vi "Drive Controller.vi"(8 "error in":errorcluster) -> ()   [LabVIEW 2017]
doc: "This VI executes continuously carrying out the current operation and responding to updates or new operation requests. It will often contain the timing or control code that is difficult to place directly in TeleOp. This VI generally opens all sensors and motors and isolates the rest of the robot code from knowing implementation details of how the operations are carried out."
uses:
  Drive Operations.ctl
  Drive Setpoints.ctl
  <vilib>/Rock Robotics/WPI/SafetyOutput/WPI_SafetyOutputConfigMenu.ctl
  Public/Documents/Cross The Road Electronics/Phoenix-LabVIEW/Motor Controller/Controls/CTRE_Phoenix_MotorControl_ControlMode.ctl
  Public/Documents/Cross The Road Electronics/Phoenix-LabVIEW/Motor Controller/Controls/CTRE_Phoenix_MotorControl_NeutralMode.ctl
  Public/Documents/Cross The Road Electronics/Phoenix-LabVIEW/Motor Controller/Controls/CTRE_Phoenix_MotorControl_FeedbackDevice.ctl
  <vilib>/Rock Robotics/WPI/RobotDrive/WPI_RobotDriveOpen4MotorWithExistingMotors.vi
  <vilib>/Rock Robotics/WPI/RobotDrive/WPI_RobotDriveOpen2MotorWithExistingMotors.vi
  <vilib>/Rock Robotics/WPI/Framework/Completion Status.ctl
panel:
  in  "Interactive Values":T1
  in  "Buttons":cluster{"Execute Cmd":bool, "Abort Cmd":bool}
  out "Command Timing":cluster{"Start Time (ms)":u32, "Iterations":i32}
  out "Status":T3
  out "Setpoints":T4(graph)
  out "Current\nCmd":string
  # "Tip: The graph shows the motor setpoints. It may also be helpful to observe inputs and sensor values.\nYou may also want to display tuning or debugging controls."
  # "Interactive Command: You may fill in the settings for a command\nand schedule it with the Execute button. You can observe and abort\nany command while fine tuning the code for the controller."
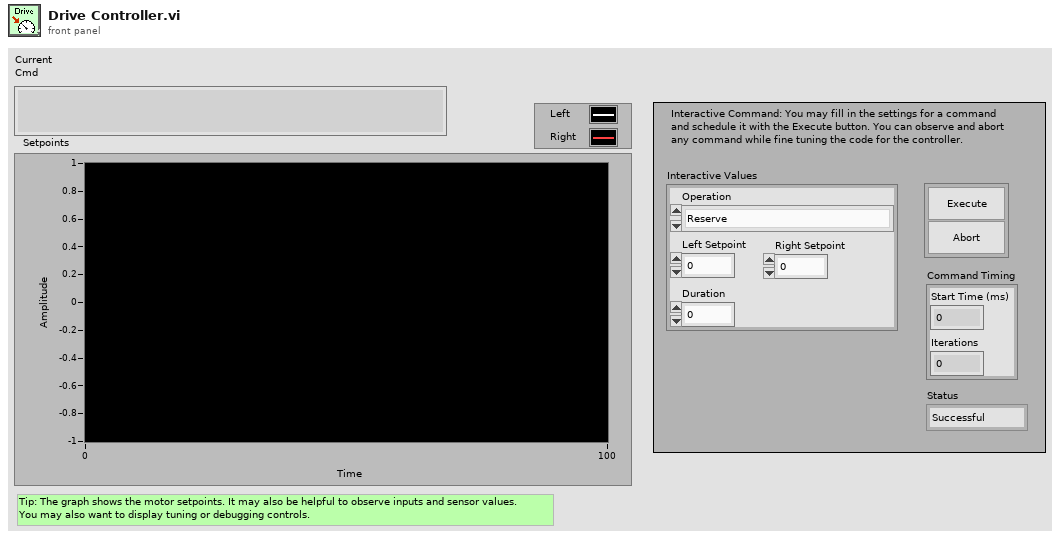
[diagram p1: front panel]
types:
  T1 = typedef "Drive Setpoints.ctl" = cluster{"Operation":T2, "Left Setpoint":dbl, "Right Setpoint":dbl, "Duration":dbl}
  T2 = typedef "Drive Operations.ctl" = enum16{"Reserve", "Read Current", "Immediate", "Drive for Time", "Drive for Distance"}
  T3 = typedef "Completion Status.ctl" = enum16{"Successful", "Aborted", "Incomplete"}
  T4 = cluster{"Left Setpoint":dbl, "Right Setpoint":dbl}
  T5 = typedef "WPI_SafetyOutputConfigMenu.ctl" = enum16{"Enable", "Disable"}
  T6 = typedef "CTRE_Phoenix_MotorControl_NeutralMode.ctl" = enum8{"EEPROMSetting", "Override to Coast", "Override to Brake"}
  T7 = typedef "CTRE_Phoenix_MotorControl_ControlMode.ctl" = u16
  T8 = typedef "CTRE_Phoenix_MotorControl_FeedbackDevice.ctl" = i8
  T9 = typedef "WPI_MotorControlDeviceRef.ctl" = cluster{"DeviceStatus":errorcluster, "Type":T10, "PWM":cluster{"PWM Channel":T11, "DeadBand":T12}, "CAN":cluster{"Device Number":u8, "SetOutput VI Ref":variant, "GetOutput VI Ref":variant, "Enable VI Ref":variant, "Disable VI Ref":variant, "Data":variant}, "Invert":bool, "DIO PWM":cluster{"PWM \"Enable\" Channel":T11, "DIOChannel":T13, "PWM Rate":dbl}}
  T10 = typedef "WPI_MotorControlType.ctl" = enum16{"PWM", "CAN", "DIO PWM"}
  T11 = typedef "FPGA_DIOPWMChannel.ctl" = enum8{"PWM 0", "PWM 1", "PWM 2", "PWM 3", "PWM 4", "PWM 5", "PWM 6", "PWM 7", "PWM 8", "PWM 9", "PWM MXP 0", "PWM MXP 1", "PWM MXP 2", "PWM MXP 3", "PWM MXP 4", "PWM MXP 5", "PWM MXP 6", "PWM MXP 7", "PWM MXP 8", "PWM MXP 9", "Invalid"}
  T12 = typedef "WPI_PWMDeadband.ctl" = cluster{"Name":string, "maxPositivePwm":i32, "minPositivePwm":i32, "centerPwm":i32, "maxNegativePwm":i32, "minNegativePwm":i32, "angularRange":u16}
  T13 = typedef "FPGA_DIOChannel.ctl" = enum8{"DIO 0", "DIO 1", "DIO 2", "DIO 3", "DIO 4", "DIO 5", "DIO 6", "DIO 7", "DIO 8", "DIO 9", "DIO MXP 0", "DIO MXP 1", "DIO MXP 2", "DIO MXP 3", "DIO MXP 4", "DIO MXP 5", "DIO MXP 6", "DIO MXP 7", "DIO MXP 8", "DIO MXP 9", "DIO MXP 10", "DIO MXP 11", "DIO MXP 12", "DIO MXP 13", "DIO MXP 14", "DIO MXP 15", "SPI Port CS1", "SPI Port CS2", "SPI Port CS3", "SPI Port MISO", "SPI Port MOSI", "Invalid"}
  T14 = typedef "WPI_RobotDriveDevRef.ctl" = cluster{"DevStatus":errorcluster, "Motors[]":T9[], "Square Inputs":bool, "Max Output":dbl}
  T15 = typedef "Command Status Info.ctl" = cluster{"Name":string, "Status":T3, "notifier out":T16}
  T16 = typedef "Completion Notifier.ctl" = refnum<notifier>
  T17 = cluster{"SubSystem Data":T1, cluster{"Start Time (ms)":u32, "Iterations":i32}, cluster{"Command Info":T15, "Description":string, "Default Command":T1, "queue out":refnum<queue>, "Subsystem Name":string}}
  T18 = cluster{"SubSystem Data":T1, cluster{"Start Time (ms)":u32, "Iterations":i32}, "Default Command Arguments":cluster{"Command Info":T15, "Description":string, "Default Command":T1, "queue out":refnum<queue>, "Subsystem Name":string}}
  T19 = cluster{"Don't move motors while reserved":dbl, "Don't move motors while reserved":dbl}
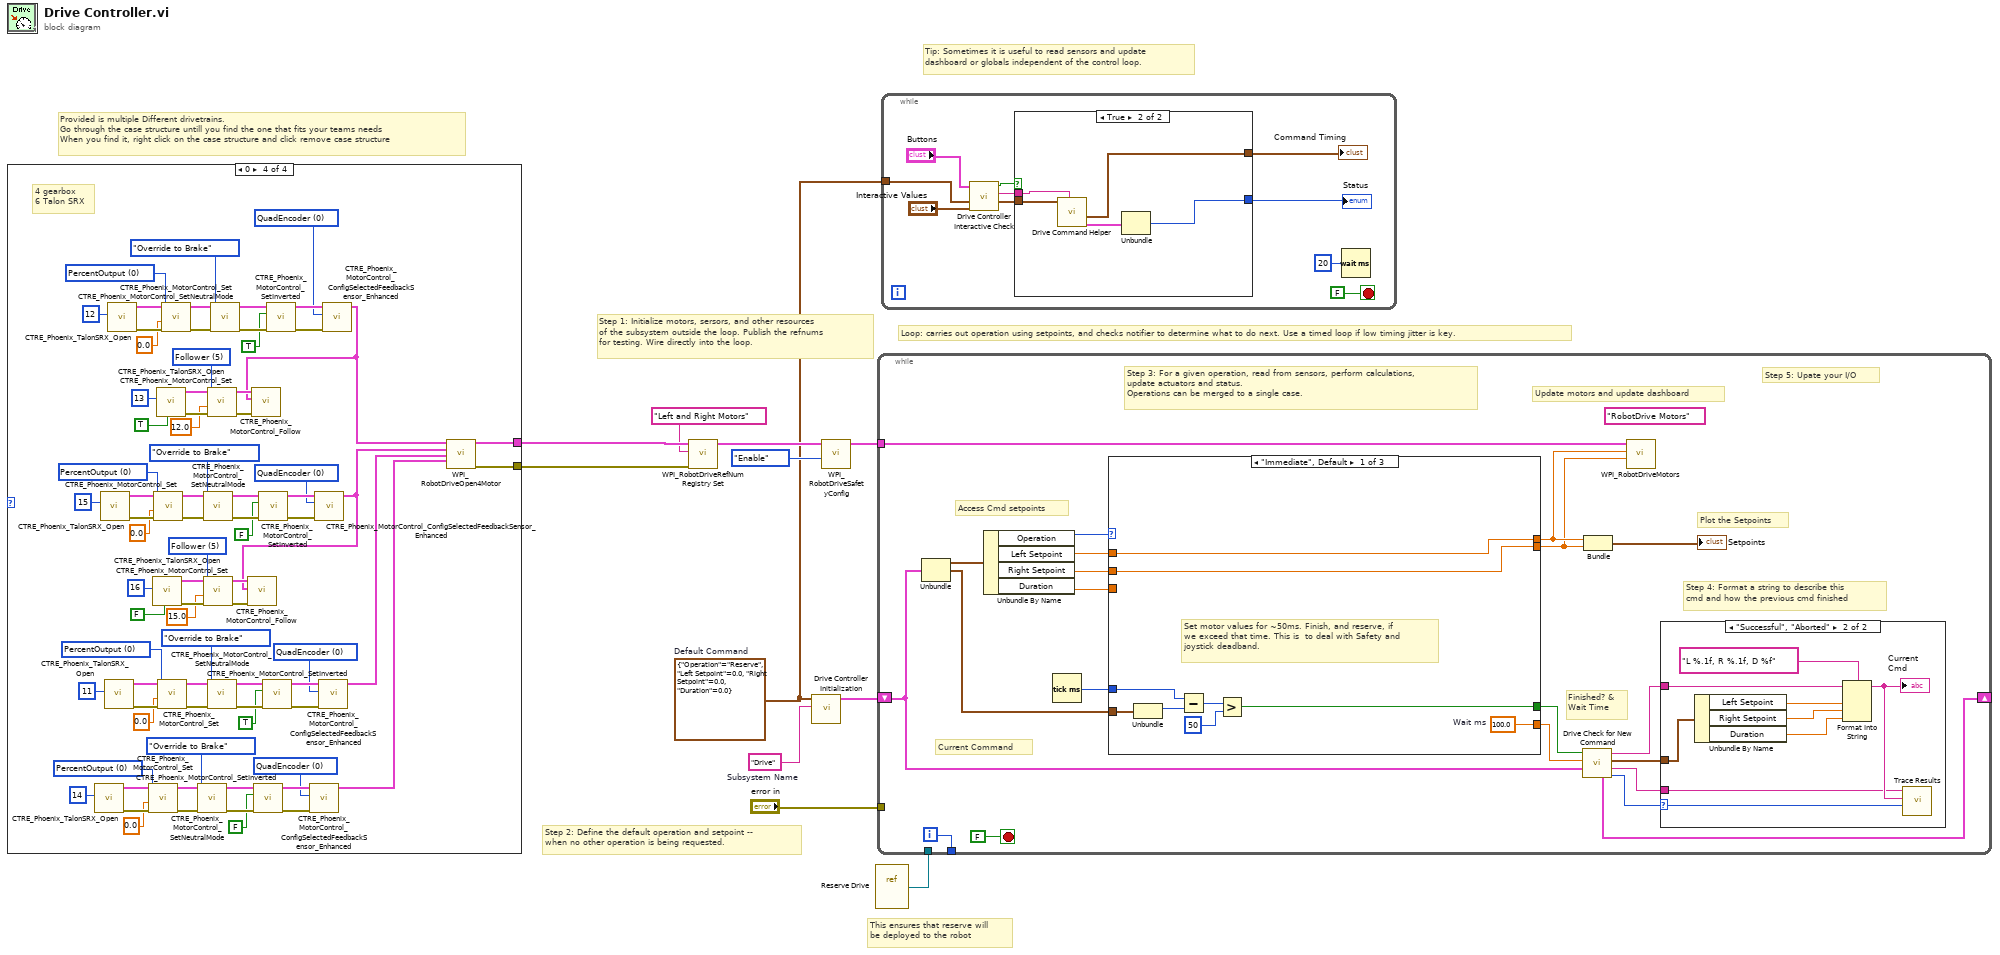
[diagram p0: block diagram]
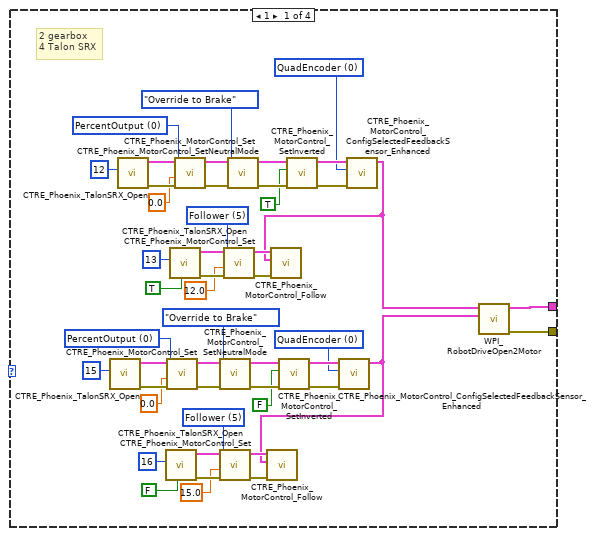
[diagram p2: hidden frame]
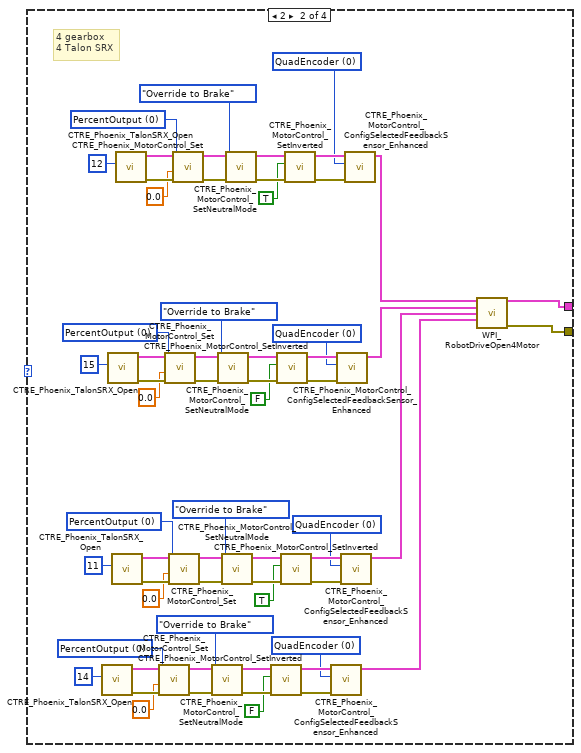
[diagram p3: hidden frame]
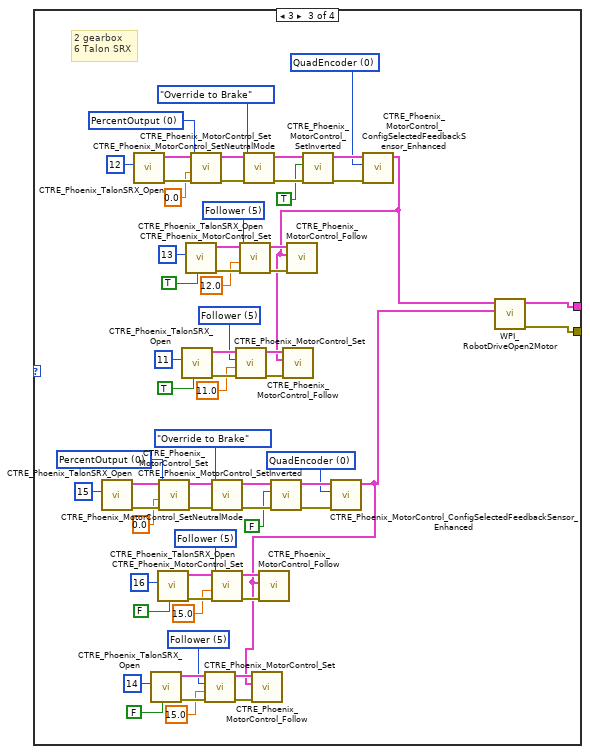
[diagram p4: hidden frame]
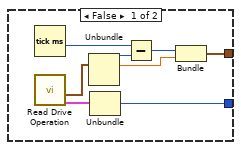
[diagram p5: hidden frame]
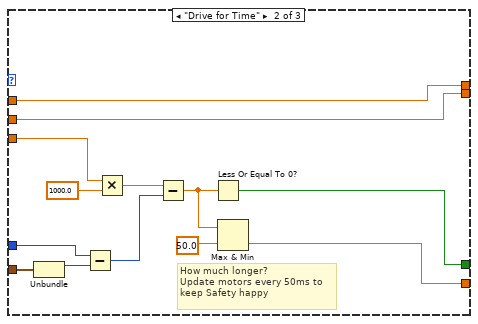
[diagram p7: hidden frame]
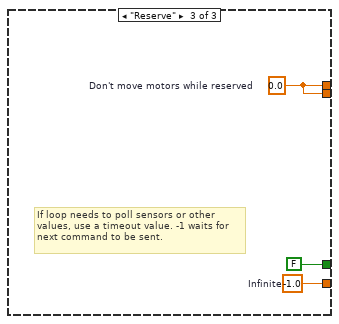
[diagram p8: hidden frame]
diagram:
  w1 = T1 {"Operation"=enum."Reserve", "Left Setpoint"=0.0, "Right Setpoint"=0.0, "Duration"=0.0}  # Default Command
  w11 = "Drive"  # Subsystem Name
  # "Provided is multiple Different drivetrains. \nGo through the case structure untill you find the one that fits your teams needs\nWhen you find it, right click on the case structure and click remove case structure"
  # "This ensures that reserve will\nbe deployed to the robot"
  # "Tip: Sometimes it is useful to read sensors and update\ndashboard or globals independent of the control loop."
  # "Step 2: Define the default operation and setpoint --\nwhen no other operation is being requested."
  # "Step 1: Initialize motors, sersors, and other resources\nof the subsystem outside the loop. Publish the refnums\nfor testing. Wire directly into the loop."
  # "Loop: carries out operation using setpoints, and checks notifier to determine what to do next. Use a timed loop if low timing jitter is key."
  n1 = case shown="0" {
    selector: _ -> [_ _ _ _]
    tunnel: [w15 w61 w141 w263] -> w10
    tunnel: [w14 w60 w140 w262] -> w8
    frame 1 {
      w21 = T7 5 items=["PercentOutput"=0, "Position"=1, "Velocity"=2, "Follower"=5, "MotionProfile"=6, "MotionMagic"=7, "MotionMagicArc"=8, "TimedPercentOutput"=9, "Disabled"=15] ("Control Mode")
      w28 = T7 5 items=["PercentOutput"=0, "Position"=1, "Velocity"=2, "Follower"=5, "MotionProfile"=6, "MotionMagic"=7, "MotionMagicArc"=8, "TimedPercentOutput"=9, "Disabled"=15] ("Control Mode")
      w32 = T8 0 items=["None"=-1, "QuadEncoder"=0, "Analog"=2, "Tachometer"=4, "Pulse Width Encoded Position"=8, "Sensor Sum (S0 + S1)"=9, "Sensor Difference (D0 - D1)"=10, "Remote Source 0"=11, "Remote Source 1"=12, "Software Emulated"=15] ("Feedback Device")
      w43 = T7 0 items=["PercentOutput"=0, "Position"=1, "Velocity"=2, "Follower"=5, "MotionProfile"=6, "MotionMagic"=7, "MotionMagicArc"=8, "TimedPercentOutput"=9, "Disabled"=15] ("Control Mode")
      w46 = T8 0 items=["None"=-1, "QuadEncoder"=0, "Analog"=2, "Tachometer"=4, "Pulse Width Encoded Position"=8, "Sensor Sum (S0 + S1)"=9, "Sensor Difference (D0 - D1)"=10, "Remote Source 0"=11, "Remote Source 1"=12, "Software Emulated"=15] ("Feedback Device")
      w57 = T7 0 items=["PercentOutput"=0, "Position"=1, "Velocity"=2, "Follower"=5, "MotionProfile"=6, "MotionMagic"=7, "MotionMagicArc"=8, "TimedPercentOutput"=9, "Disabled"=15] ("Control Mode")
      # "2 gearbox\n4 Talon SRX"
      n2 = call "CTRE_Phoenix_TalonSRX_Open.vi"("Device Number"=u8 15) -> ("error out"=w45:errorcluster, "CAN Talon SRX Ref"=w44:T9)  [unwired: 9 in]
      n3 = call "CTRE_Phoenix_TalonSRX_Open.vi"("Device Number"=u8 12) -> ("error out"=w59:errorcluster, "CAN Talon SRX Ref"=w58:T9)  [unwired: 9 in]
      n4 = call "CTRE_Phoenix_TalonSRX_Open.vi"("Invert"=FALSE, "Device Number"=u8 16) -> ("error out"=w23:errorcluster, "CAN Talon SRX Ref"=w22:T9)  [unwired: 8 in]
      n5 = call "CTRE_Phoenix_MotorControl_Set.vi"("error in (no error)"=w45, "Output"=0.0, "Control Mode"=w43, "PhoenixMotorControlDevRef"=w44) -> ("error out"=w40:errorcluster, "PhoenixMotorControlDevRef"=w39:T9)  [unwired: 6 in]
      n6 = call "CTRE_Phoenix_TalonSRX_Open.vi"("Invert"=TRUE, "Device Number"=u8 13) -> ("error out"=w30:errorcluster, "CAN Talon SRX Ref"=w29:T9)  [unwired: 8 in]
      n7 = call "CTRE_Phoenix_MotorControl_Set.vi"("error in (no error)"=w59, "Output"=0.0, "Control Mode"=w57, "PhoenixMotorControlDevRef"=w58) -> ("error out"=w54:errorcluster, "PhoenixMotorControlDevRef"=w53:T9)  [unwired: 6 in]
      n8 = call "CTRE_Phoenix_MotorControl_SetNeutralMode.vi"("error in (no error)"=w40, "Motor Control Neutral Mode"=CTRE_Phoenix_MotorControl_NeutralMode."Override to Brake", "PhoenixMotorControlDevRef"=w39) -> ("error out"=w37:errorcluster, "PhoenixMotorControlDevRef"=w36:T9)  [unwired: 7 in]
      n9 = call "CTRE_Phoenix_MotorControl_Set.vi"("error in (no error)"=w23, "Output"=15.0, "Control Mode"=w21, "PhoenixMotorControlDevRef"=w22) -> ("error out"=w19:errorcluster, "PhoenixMotorControlDevRef"=w18:T9)  [unwired: 6 in]
      n10 = call "CTRE_Phoenix_MotorControl_Set.vi"("error in (no error)"=w30, "Output"=12.0, "Control Mode"=w28, "PhoenixMotorControlDevRef"=w29) -> ("error out"=w26:errorcluster, "PhoenixMotorControlDevRef"=w25:T9)  [unwired: 6 in]
      n11 = call "CTRE_Phoenix_MotorControl_SetNeutralMode.vi"("error in (no error)"=w54, "Motor Control Neutral Mode"=CTRE_Phoenix_MotorControl_NeutralMode."Override to Brake", "PhoenixMotorControlDevRef"=w53) -> ("error out"=w51:errorcluster, "PhoenixMotorControlDevRef"=w50:T9)  [unwired: 7 in]
      n12 = call "CTRE_Phoenix_MotorControl_SetInverted.vi"("error in (no error)"=w37, "Invert?"=FALSE, "PhoenixMotorControlDevRef"=w36) -> ("error out"=w34:errorcluster, "PhoenixMotorControlDevRef"=w33:T9)  [unwired: 7 in]
      n13 = call "CTRE_Phoenix_MotorControl_SetInverted.vi"("error in (no error)"=w51, "Invert?"=TRUE, "PhoenixMotorControlDevRef"=w50) -> ("error out"=w48:errorcluster, "PhoenixMotorControlDevRef"=w47:T9)  [unwired: 7 in]
      n14 = call "CTRE_Phoenix_MotorControl_ConfigSelectedFeedbackSensor_Enhanced.vi"("error in (no error)"=w34, "Feedback Device"=w32, "PhoenixMotorControlDevRef"=w33) -> ("PhoenixMotorControlDevRef"=w12:T9)  [unwired: 7 in, 1 out]
      n15 = call "CTRE_Phoenix_MotorControl_Follow.vi"("error in (no error)"=w19, "Master Controller to Follow"=w12, "PhoenixMotorControlDevRef"=w18) -> ()  [unwired: 7 in, 2 out]
      n16 = call "CTRE_Phoenix_MotorControl_ConfigSelectedFeedbackSensor_Enhanced.vi"("error in (no error)"=w48, "Feedback Device"=w46, "PhoenixMotorControlDevRef"=w47) -> ("PhoenixMotorControlDevRef"=w13:T9)  [unwired: 7 in, 1 out]
      n17 = call "CTRE_Phoenix_MotorControl_Follow.vi"("error in (no error)"=w26, "Master Controller to Follow"=w13, "PhoenixMotorControlDevRef"=w25) -> ()  [unwired: 7 in, 2 out]
      n18 = call-poly <vilib>:"WPI_RobotDriveOpen2Motor.vi"("Right Motor Dev Ref"=w12, "Left Motor Dev Ref"=w13) -> ("error out"=w14:errorcluster, "RobotDriveDevRef"=w15:T14)  [unwired: 8 in]
    }
    frame 2 {
      w66 = T8 0 items=["None"=-1, "QuadEncoder"=0, "Analog"=2, "Tachometer"=4, "Pulse Width Encoded Position"=8, "Sensor Sum (S0 + S1)"=9, "Sensor Difference (D0 - D1)"=10, "Remote Source 0"=11, "Remote Source 1"=12, "Software Emulated"=15] ("Feedback Device")
      w77 = T7 0 items=["PercentOutput"=0, "Position"=1, "Velocity"=2, "Follower"=5, "MotionProfile"=6, "MotionMagic"=7, "MotionMagicArc"=8, "TimedPercentOutput"=9, "Disabled"=15] ("Control Mode")
      w80 = T8 0 items=["None"=-1, "QuadEncoder"=0, "Analog"=2, "Tachometer"=4, "Pulse Width Encoded Position"=8, "Sensor Sum (S0 + S1)"=9, "Sensor Difference (D0 - D1)"=10, "Remote Source 0"=11, "Remote Source 1"=12, "Software Emulated"=15] ("Feedback Device")
      w91 = T7 0 items=["PercentOutput"=0, "Position"=1, "Velocity"=2, "Follower"=5, "MotionProfile"=6, "MotionMagic"=7, "MotionMagicArc"=8, "TimedPercentOutput"=9, "Disabled"=15] ("Control Mode")
      w94 = T8 0 items=["None"=-1, "QuadEncoder"=0, "Analog"=2, "Tachometer"=4, "Pulse Width Encoded Position"=8, "Sensor Sum (S0 + S1)"=9, "Sensor Difference (D0 - D1)"=10, "Remote Source 0"=11, "Remote Source 1"=12, "Software Emulated"=15] ("Feedback Device")
      w105 = T7 0 items=["PercentOutput"=0, "Position"=1, "Velocity"=2, "Follower"=5, "MotionProfile"=6, "MotionMagic"=7, "MotionMagicArc"=8, "TimedPercentOutput"=9, "Disabled"=15] ("Control Mode")
      w108 = T8 0 items=["None"=-1, "QuadEncoder"=0, "Analog"=2, "Tachometer"=4, "Pulse Width Encoded Position"=8, "Sensor Sum (S0 + S1)"=9, "Sensor Difference (D0 - D1)"=10, "Remote Source 0"=11, "Remote Source 1"=12, "Software Emulated"=15] ("Feedback Device")
      w119 = T7 0 items=["PercentOutput"=0, "Position"=1, "Velocity"=2, "Follower"=5, "MotionProfile"=6, "MotionMagic"=7, "MotionMagicArc"=8, "TimedPercentOutput"=9, "Disabled"=15] ("Control Mode")
      # "4 gearbox\n4 Talon SRX"
      n19 = call "CTRE_Phoenix_TalonSRX_Open.vi"("Device Number"=u8 14) -> ("error out"=w79:errorcluster, "CAN Talon SRX Ref"=w78:T9)  [unwired: 9 in]
      n20 = call "CTRE_Phoenix_TalonSRX_Open.vi"("Device Number"=u8 15) -> ("error out"=w107:errorcluster, "CAN Talon SRX Ref"=w106:T9)  [unwired: 9 in]
      n21 = call "CTRE_Phoenix_TalonSRX_Open.vi"("Device Number"=u8 11) -> ("error out"=w93:errorcluster, "CAN Talon SRX Ref"=w92:T9)  [unwired: 9 in]
      n22 = call "CTRE_Phoenix_TalonSRX_Open.vi"("Device Number"=u8 12) -> ("error out"=w121:errorcluster, "CAN Talon SRX Ref"=w120:T9)  [unwired: 9 in]
      n23 = call "CTRE_Phoenix_MotorControl_Set.vi"("error in (no error)"=w79, "Output"=0.0, "Control Mode"=w77, "PhoenixMotorControlDevRef"=w78) -> ("error out"=w74:errorcluster, "PhoenixMotorControlDevRef"=w73:T9)  [unwired: 6 in]
      n24 = call "CTRE_Phoenix_MotorControl_Set.vi"("error in (no error)"=w107, "Output"=0.0, "Control Mode"=w105, "PhoenixMotorControlDevRef"=w106) -> ("error out"=w102:errorcluster, "PhoenixMotorControlDevRef"=w101:T9)  [unwired: 6 in]
      n25 = call "CTRE_Phoenix_MotorControl_Set.vi"("error in (no error)"=w93, "Output"=0.0, "Control Mode"=w91, "PhoenixMotorControlDevRef"=w92) -> ("error out"=w88:errorcluster, "PhoenixMotorControlDevRef"=w87:T9)  [unwired: 6 in]
      n26 = call "CTRE_Phoenix_MotorControl_Set.vi"("error in (no error)"=w121, "Output"=0.0, "Control Mode"=w119, "PhoenixMotorControlDevRef"=w120) -> ("error out"=w116:errorcluster, "PhoenixMotorControlDevRef"=w115:T9)  [unwired: 6 in]
      n27 = call "CTRE_Phoenix_MotorControl_SetNeutralMode.vi"("error in (no error)"=w74, "Motor Control Neutral Mode"=CTRE_Phoenix_MotorControl_NeutralMode."Override to Brake", "PhoenixMotorControlDevRef"=w73) -> ("error out"=w71:errorcluster, "PhoenixMotorControlDevRef"=w70:T9)  [unwired: 7 in]
      n28 = call "CTRE_Phoenix_MotorControl_SetNeutralMode.vi"("error in (no error)"=w102, "Motor Control Neutral Mode"=CTRE_Phoenix_MotorControl_NeutralMode."Override to Brake", "PhoenixMotorControlDevRef"=w101) -> ("error out"=w99:errorcluster, "PhoenixMotorControlDevRef"=w98:T9)  [unwired: 7 in]
      n29 = call "CTRE_Phoenix_MotorControl_SetNeutralMode.vi"("error in (no error)"=w88, "Motor Control Neutral Mode"=CTRE_Phoenix_MotorControl_NeutralMode."Override to Brake", "PhoenixMotorControlDevRef"=w87) -> ("error out"=w85:errorcluster, "PhoenixMotorControlDevRef"=w84:T9)  [unwired: 7 in]
      n30 = call "CTRE_Phoenix_MotorControl_SetNeutralMode.vi"("error in (no error)"=w116, "Motor Control Neutral Mode"=CTRE_Phoenix_MotorControl_NeutralMode."Override to Brake", "PhoenixMotorControlDevRef"=w115) -> ("error out"=w113:errorcluster, "PhoenixMotorControlDevRef"=w112:T9)  [unwired: 7 in]
      n31 = call "CTRE_Phoenix_MotorControl_SetInverted.vi"("error in (no error)"=w71, "Invert?"=FALSE, "PhoenixMotorControlDevRef"=w70) -> ("error out"=w68:errorcluster, "PhoenixMotorControlDevRef"=w67:T9)  [unwired: 7 in]
      n32 = call "CTRE_Phoenix_MotorControl_SetInverted.vi"("error in (no error)"=w99, "Invert?"=FALSE, "PhoenixMotorControlDevRef"=w98) -> ("error out"=w96:errorcluster, "PhoenixMotorControlDevRef"=w95:T9)  [unwired: 7 in]
      n33 = call "CTRE_Phoenix_MotorControl_SetInverted.vi"("error in (no error)"=w85, "Invert?"=TRUE, "PhoenixMotorControlDevRef"=w84) -> ("error out"=w82:errorcluster, "PhoenixMotorControlDevRef"=w81:T9)  [unwired: 7 in]
      n34 = call "CTRE_Phoenix_MotorControl_SetInverted.vi"("error in (no error)"=w113, "Invert?"=TRUE, "PhoenixMotorControlDevRef"=w112) -> ("error out"=w110:errorcluster, "PhoenixMotorControlDevRef"=w109:T9)  [unwired: 7 in]
      n35 = call "CTRE_Phoenix_MotorControl_ConfigSelectedFeedbackSensor_Enhanced.vi"("error in (no error)"=w68, "Feedback Device"=w66, "PhoenixMotorControlDevRef"=w67) -> ("PhoenixMotorControlDevRef"=w62:T9)  [unwired: 7 in, 1 out]
      n36 = call "CTRE_Phoenix_MotorControl_ConfigSelectedFeedbackSensor_Enhanced.vi"("error in (no error)"=w96, "Feedback Device"=w94, "PhoenixMotorControlDevRef"=w95) -> ("PhoenixMotorControlDevRef"=w64:T9)  [unwired: 7 in, 1 out]
      n37 = call "CTRE_Phoenix_MotorControl_ConfigSelectedFeedbackSensor_Enhanced.vi"("error in (no error)"=w82, "Feedback Device"=w80, "PhoenixMotorControlDevRef"=w81) -> ("PhoenixMotorControlDevRef"=w63:T9)  [unwired: 7 in, 1 out]
      n38 = call "CTRE_Phoenix_MotorControl_ConfigSelectedFeedbackSensor_Enhanced.vi"("error in (no error)"=w110, "Feedback Device"=w108, "PhoenixMotorControlDevRef"=w109) -> ("PhoenixMotorControlDevRef"=w65:T9)  [unwired: 7 in, 1 out]
      n39 = call-poly <vilib>:"WPI_RobotDriveOpen4Motor.vi"("Rear Left Motor Dev Ref"=w65, "Rear Right Motor Dev Ref"=w64, "Front Left Motor Dev Ref"=w63, "Front Right Motor Dev Ref"=w62) -> ("RobotDriveDevRef"=w61:T14, "error out"=w60:errorcluster)  [unwired: 10 in]
    }
    frame 3 {
      w124 = T7 5 items=["PercentOutput"=0, "Position"=1, "Velocity"=2, "Follower"=5, "MotionProfile"=6, "MotionMagic"=7, "MotionMagicArc"=8, "TimedPercentOutput"=9, "Disabled"=15] ("Control Mode")
      w125 = T7 5 items=["PercentOutput"=0, "Position"=1, "Velocity"=2, "Follower"=5, "MotionProfile"=6, "MotionMagic"=7, "MotionMagicArc"=8, "TimedPercentOutput"=9, "Disabled"=15] ("Control Mode")
      w147 = T7 5 items=["PercentOutput"=0, "Position"=1, "Velocity"=2, "Follower"=5, "MotionProfile"=6, "MotionMagic"=7, "MotionMagicArc"=8, "TimedPercentOutput"=9, "Disabled"=15] ("Control Mode")
      w154 = T7 5 items=["PercentOutput"=0, "Position"=1, "Velocity"=2, "Follower"=5, "MotionProfile"=6, "MotionMagic"=7, "MotionMagicArc"=8, "TimedPercentOutput"=9, "Disabled"=15] ("Control Mode")
      w158 = T8 0 items=["None"=-1, "QuadEncoder"=0, "Analog"=2, "Tachometer"=4, "Pulse Width Encoded Position"=8, "Sensor Sum (S0 + S1)"=9, "Sensor Difference (D0 - D1)"=10, "Remote Source 0"=11, "Remote Source 1"=12, "Software Emulated"=15] ("Feedback Device")
      w169 = T7 0 items=["PercentOutput"=0, "Position"=1, "Velocity"=2, "Follower"=5, "MotionProfile"=6, "MotionMagic"=7, "MotionMagicArc"=8, "TimedPercentOutput"=9, "Disabled"=15] ("Control Mode")
      w172 = T8 0 items=["None"=-1, "QuadEncoder"=0, "Analog"=2, "Tachometer"=4, "Pulse Width Encoded Position"=8, "Sensor Sum (S0 + S1)"=9, "Sensor Difference (D0 - D1)"=10, "Remote Source 0"=11, "Remote Source 1"=12, "Software Emulated"=15] ("Feedback Device")
      w183 = T7 0 items=["PercentOutput"=0, "Position"=1, "Velocity"=2, "Follower"=5, "MotionProfile"=6, "MotionMagic"=7, "MotionMagicArc"=8, "TimedPercentOutput"=9, "Disabled"=15] ("Control Mode")
      # "2 gearbox\n6 Talon SRX"
      n40 = call "CTRE_Phoenix_TalonSRX_Open.vi"("Device Number"=u8 15) -> ("error out"=w171:errorcluster, "CAN Talon SRX Ref"=w170:T9)  [unwired: 9 in]
      n41 = call "CTRE_Phoenix_TalonSRX_Open.vi"("Device Number"=u8 12) -> ("error out"=w185:errorcluster, "CAN Talon SRX Ref"=w184:T9)  [unwired: 9 in]
      n42 = call "CTRE_Phoenix_TalonSRX_Open.vi"("Invert"=FALSE, "Device Number"=u8 14) -> ("error out"=w138:errorcluster, "CAN Talon SRX Ref"=w137:T9)  [unwired: 8 in]
      n43 = call "CTRE_Phoenix_TalonSRX_Open.vi"("Invert"=FALSE, "Device Number"=u8 16) -> ("error out"=w149:errorcluster, "CAN Talon SRX Ref"=w148:T9)  [unwired: 8 in]
      n44 = call "CTRE_Phoenix_MotorControl_Set.vi"("error in (no error)"=w171, "Output"=0.0, "Control Mode"=w169, "PhoenixMotorControlDevRef"=w170) -> ("error out"=w166:errorcluster, "PhoenixMotorControlDevRef"=w165:T9)  [unwired: 6 in]
      n45 = call "CTRE_Phoenix_TalonSRX_Open.vi"("Invert"=TRUE, "Device Number"=u8 11) -> ("error out"=w131:errorcluster, "CAN Talon SRX Ref"=w130:T9)  [unwired: 8 in]
      n46 = call "CTRE_Phoenix_TalonSRX_Open.vi"("Invert"=TRUE, "Device Number"=u8 13) -> ("error out"=w156:errorcluster, "CAN Talon SRX Ref"=w155:T9)  [unwired: 8 in]
      n47 = call "CTRE_Phoenix_MotorControl_Set.vi"("error in (no error)"=w185, "Output"=0.0, "Control Mode"=w183, "PhoenixMotorControlDevRef"=w184) -> ("error out"=w180:errorcluster, "PhoenixMotorControlDevRef"=w179:T9)  [unwired: 6 in]
      n48 = call "CTRE_Phoenix_MotorControl_Set.vi"("error in (no error)"=w138, "Output"=15.0, "Control Mode"=w125, "PhoenixMotorControlDevRef"=w137) -> ("error out"=w135:errorcluster, "PhoenixMotorControlDevRef"=w134:T9)  [unwired: 6 in]
      n49 = call "CTRE_Phoenix_MotorControl_SetNeutralMode.vi"("error in (no error)"=w166, "Motor Control Neutral Mode"=CTRE_Phoenix_MotorControl_NeutralMode."Override to Brake", "PhoenixMotorControlDevRef"=w165) -> ("error out"=w163:errorcluster, "PhoenixMotorControlDevRef"=w162:T9)  [unwired: 7 in]
      n50 = call "CTRE_Phoenix_MotorControl_Set.vi"("error in (no error)"=w149, "Output"=15.0, "Control Mode"=w147, "PhoenixMotorControlDevRef"=w148) -> ("error out"=w145:errorcluster, "PhoenixMotorControlDevRef"=w144:T9)  [unwired: 6 in]
      n51 = call "CTRE_Phoenix_MotorControl_Set.vi"("error in (no error)"=w131, "Output"=11.0, "Control Mode"=w124, "PhoenixMotorControlDevRef"=w130) -> ("error out"=w128:errorcluster, "PhoenixMotorControlDevRef"=w127:T9)  [unwired: 6 in]
      n52 = call "CTRE_Phoenix_MotorControl_Set.vi"("error in (no error)"=w156, "Output"=12.0, "Control Mode"=w154, "PhoenixMotorControlDevRef"=w155) -> ("error out"=w152:errorcluster, "PhoenixMotorControlDevRef"=w151:T9)  [unwired: 6 in]
      n53 = call "CTRE_Phoenix_MotorControl_SetNeutralMode.vi"("error in (no error)"=w180, "Motor Control Neutral Mode"=CTRE_Phoenix_MotorControl_NeutralMode."Override to Brake", "PhoenixMotorControlDevRef"=w179) -> ("error out"=w177:errorcluster, "PhoenixMotorControlDevRef"=w176:T9)  [unwired: 7 in]
      n54 = call "CTRE_Phoenix_MotorControl_SetInverted.vi"("error in (no error)"=w163, "Invert?"=FALSE, "PhoenixMotorControlDevRef"=w162) -> ("error out"=w160:errorcluster, "PhoenixMotorControlDevRef"=w159:T9)  [unwired: 7 in]
      n55 = call "CTRE_Phoenix_MotorControl_SetInverted.vi"("error in (no error)"=w177, "Invert?"=TRUE, "PhoenixMotorControlDevRef"=w176) -> ("error out"=w174:errorcluster, "PhoenixMotorControlDevRef"=w173:T9)  [unwired: 7 in]
      n56 = call "CTRE_Phoenix_MotorControl_ConfigSelectedFeedbackSensor_Enhanced.vi"("error in (no error)"=w160, "Feedback Device"=w158, "PhoenixMotorControlDevRef"=w159) -> ("PhoenixMotorControlDevRef"=w122:T9)  [unwired: 7 in, 1 out]
      n57 = call "CTRE_Phoenix_MotorControl_Follow.vi"("error in (no error)"=w135, "Master Controller to Follow"=w122, "PhoenixMotorControlDevRef"=w134) -> ()  [unwired: 7 in, 2 out]
      n58 = call "CTRE_Phoenix_MotorControl_Follow.vi"("error in (no error)"=w145, "Master Controller to Follow"=w122, "PhoenixMotorControlDevRef"=w144) -> ()  [unwired: 7 in, 2 out]
      n59 = call "CTRE_Phoenix_MotorControl_ConfigSelectedFeedbackSensor_Enhanced.vi"("error in (no error)"=w174, "Feedback Device"=w172, "PhoenixMotorControlDevRef"=w173) -> ("PhoenixMotorControlDevRef"=w123:T9)  [unwired: 7 in, 1 out]
      n60 = call "CTRE_Phoenix_MotorControl_Follow.vi"("error in (no error)"=w128, "Master Controller to Follow"=w123, "PhoenixMotorControlDevRef"=w127) -> ()  [unwired: 7 in, 2 out]
      n61 = call "CTRE_Phoenix_MotorControl_Follow.vi"("error in (no error)"=w152, "Master Controller to Follow"=w123, "PhoenixMotorControlDevRef"=w151) -> ()  [unwired: 7 in, 2 out]
      n62 = call-poly <vilib>:"WPI_RobotDriveOpen2Motor.vi"("Right Motor Dev Ref"=w122, "Left Motor Dev Ref"=w123) -> ("error out"=w140:errorcluster, "RobotDriveDevRef"=w141:T14)  [unwired: 8 in]
    }
    frame 0 {
      w195 = T7 5 items=["PercentOutput"=0, "Position"=1, "Velocity"=2, "Follower"=5, "MotionProfile"=6, "MotionMagic"=7, "MotionMagicArc"=8, "TimedPercentOutput"=9, "Disabled"=15] ("Control Mode")
      w202 = T7 5 items=["PercentOutput"=0, "Position"=1, "Velocity"=2, "Follower"=5, "MotionProfile"=6, "MotionMagic"=7, "MotionMagicArc"=8, "TimedPercentOutput"=9, "Disabled"=15] ("Control Mode")
      w206 = T8 0 items=["None"=-1, "QuadEncoder"=0, "Analog"=2, "Tachometer"=4, "Pulse Width Encoded Position"=8, "Sensor Sum (S0 + S1)"=9, "Sensor Difference (D0 - D1)"=10, "Remote Source 0"=11, "Remote Source 1"=12, "Software Emulated"=15] ("Feedback Device")
      w217 = T7 0 items=["PercentOutput"=0, "Position"=1, "Velocity"=2, "Follower"=5, "MotionProfile"=6, "MotionMagic"=7, "MotionMagicArc"=8, "TimedPercentOutput"=9, "Disabled"=15] ("Control Mode")
      w220 = T8 0 items=["None"=-1, "QuadEncoder"=0, "Analog"=2, "Tachometer"=4, "Pulse Width Encoded Position"=8, "Sensor Sum (S0 + S1)"=9, "Sensor Difference (D0 - D1)"=10, "Remote Source 0"=11, "Remote Source 1"=12, "Software Emulated"=15] ("Feedback Device")
      w231 = T7 0 items=["PercentOutput"=0, "Position"=1, "Velocity"=2, "Follower"=5, "MotionProfile"=6, "MotionMagic"=7, "MotionMagicArc"=8, "TimedPercentOutput"=9, "Disabled"=15] ("Control Mode")
      w234 = T8 0 items=["None"=-1, "QuadEncoder"=0, "Analog"=2, "Tachometer"=4, "Pulse Width Encoded Position"=8, "Sensor Sum (S0 + S1)"=9, "Sensor Difference (D0 - D1)"=10, "Remote Source 0"=11, "Remote Source 1"=12, "Software Emulated"=15] ("Feedback Device")
      w245 = T7 0 items=["PercentOutput"=0, "Position"=1, "Velocity"=2, "Follower"=5, "MotionProfile"=6, "MotionMagic"=7, "MotionMagicArc"=8, "TimedPercentOutput"=9, "Disabled"=15] ("Control Mode")
      w248 = T8 0 items=["None"=-1, "QuadEncoder"=0, "Analog"=2, "Tachometer"=4, "Pulse Width Encoded Position"=8, "Sensor Sum (S0 + S1)"=9, "Sensor Difference (D0 - D1)"=10, "Remote Source 0"=11, "Remote Source 1"=12, "Software Emulated"=15] ("Feedback Device")
      w259 = T7 0 items=["PercentOutput"=0, "Position"=1, "Velocity"=2, "Follower"=5, "MotionProfile"=6, "MotionMagic"=7, "MotionMagicArc"=8, "TimedPercentOutput"=9, "Disabled"=15] ("Control Mode")
      # "4 gearbox\n6 Talon SRX"
      n63 = call "CTRE_Phoenix_TalonSRX_Open.vi"("Device Number"=u8 14) -> ("error out"=w219:errorcluster, "CAN Talon SRX Ref"=w218:T9)  [unwired: 9 in]
      n64 = call "CTRE_Phoenix_TalonSRX_Open.vi"("Device Number"=u8 15) -> ("error out"=w247:errorcluster, "CAN Talon SRX Ref"=w246:T9)  [unwired: 9 in]
      n65 = call "CTRE_Phoenix_TalonSRX_Open.vi"("Device Number"=u8 11) -> ("error out"=w233:errorcluster, "CAN Talon SRX Ref"=w232:T9)  [unwired: 9 in]
      n66 = call "CTRE_Phoenix_TalonSRX_Open.vi"("Device Number"=u8 12) -> ("error out"=w261:errorcluster, "CAN Talon SRX Ref"=w260:T9)  [unwired: 9 in]
      n67 = call "CTRE_Phoenix_MotorControl_Set.vi"("error in (no error)"=w219, "Output"=0.0, "Control Mode"=w217, "PhoenixMotorControlDevRef"=w218) -> ("error out"=w214:errorcluster, "PhoenixMotorControlDevRef"=w213:T9)  [unwired: 6 in]
      n68 = call "CTRE_Phoenix_TalonSRX_Open.vi"("Invert"=FALSE, "Device Number"=u8 16) -> ("error out"=w197:errorcluster, "CAN Talon SRX Ref"=w196:T9)  [unwired: 8 in]
      n69 = call "CTRE_Phoenix_MotorControl_Set.vi"("error in (no error)"=w247, "Output"=0.0, "Control Mode"=w245, "PhoenixMotorControlDevRef"=w246) -> ("error out"=w242:errorcluster, "PhoenixMotorControlDevRef"=w241:T9)  [unwired: 6 in]
      n70 = call "CTRE_Phoenix_TalonSRX_Open.vi"("Invert"=TRUE, "Device Number"=u8 13) -> ("error out"=w204:errorcluster, "CAN Talon SRX Ref"=w203:T9)  [unwired: 8 in]
      n71 = call "CTRE_Phoenix_MotorControl_Set.vi"("error in (no error)"=w233, "Output"=0.0, "Control Mode"=w231, "PhoenixMotorControlDevRef"=w232) -> ("error out"=w228:errorcluster, "PhoenixMotorControlDevRef"=w227:T9)  [unwired: 6 in]
      n72 = call "CTRE_Phoenix_MotorControl_Set.vi"("error in (no error)"=w261, "Output"=0.0, "Control Mode"=w259, "PhoenixMotorControlDevRef"=w260) -> ("error out"=w256:errorcluster, "PhoenixMotorControlDevRef"=w255:T9)  [unwired: 6 in]
      n73 = call "CTRE_Phoenix_MotorControl_SetNeutralMode.vi"("error in (no error)"=w214, "Motor Control Neutral Mode"=CTRE_Phoenix_MotorControl_NeutralMode."Override to Brake", "PhoenixMotorControlDevRef"=w213) -> ("error out"=w211:errorcluster, "PhoenixMotorControlDevRef"=w210:T9)  [unwired: 7 in]
      n74 = call "CTRE_Phoenix_MotorControl_SetNeutralMode.vi"("error in (no error)"=w242, "Motor Control Neutral Mode"=CTRE_Phoenix_MotorControl_NeutralMode."Override to Brake", "PhoenixMotorControlDevRef"=w241) -> ("error out"=w239:errorcluster, "PhoenixMotorControlDevRef"=w238:T9)  [unwired: 7 in]
      n75 = call "CTRE_Phoenix_MotorControl_Set.vi"("error in (no error)"=w197, "Output"=15.0, "Control Mode"=w195, "PhoenixMotorControlDevRef"=w196) -> ("error out"=w193:errorcluster, "PhoenixMotorControlDevRef"=w192:T9)  [unwired: 6 in]
      n76 = call "CTRE_Phoenix_MotorControl_Set.vi"("error in (no error)"=w204, "Output"=12.0, "Control Mode"=w202, "PhoenixMotorControlDevRef"=w203) -> ("error out"=w200:errorcluster, "PhoenixMotorControlDevRef"=w199:T9)  [unwired: 6 in]
      n77 = call "CTRE_Phoenix_MotorControl_SetNeutralMode.vi"("error in (no error)"=w228, "Motor Control Neutral Mode"=CTRE_Phoenix_MotorControl_NeutralMode."Override to Brake", "PhoenixMotorControlDevRef"=w227) -> ("error out"=w225:errorcluster, "PhoenixMotorControlDevRef"=w224:T9)  [unwired: 7 in]
      n78 = call "CTRE_Phoenix_MotorControl_SetNeutralMode.vi"("error in (no error)"=w256, "Motor Control Neutral Mode"=CTRE_Phoenix_MotorControl_NeutralMode."Override to Brake", "PhoenixMotorControlDevRef"=w255) -> ("error out"=w253:errorcluster, "PhoenixMotorControlDevRef"=w252:T9)  [unwired: 7 in]
      n79 = call "CTRE_Phoenix_MotorControl_SetInverted.vi"("error in (no error)"=w211, "Invert?"=FALSE, "PhoenixMotorControlDevRef"=w210) -> ("error out"=w208:errorcluster, "PhoenixMotorControlDevRef"=w207:T9)  [unwired: 7 in]
      n80 = call "CTRE_Phoenix_MotorControl_SetInverted.vi"("error in (no error)"=w239, "Invert?"=FALSE, "PhoenixMotorControlDevRef"=w238) -> ("error out"=w236:errorcluster, "PhoenixMotorControlDevRef"=w235:T9)  [unwired: 7 in]
      n81 = call "CTRE_Phoenix_MotorControl_SetInverted.vi"("error in (no error)"=w225, "Invert?"=TRUE, "PhoenixMotorControlDevRef"=w224) -> ("error out"=w222:errorcluster, "PhoenixMotorControlDevRef"=w221:T9)  [unwired: 7 in]
      n82 = call "CTRE_Phoenix_MotorControl_SetInverted.vi"("error in (no error)"=w253, "Invert?"=TRUE, "PhoenixMotorControlDevRef"=w252) -> ("error out"=w250:errorcluster, "PhoenixMotorControlDevRef"=w249:T9)  [unwired: 7 in]
      n83 = call "CTRE_Phoenix_MotorControl_ConfigSelectedFeedbackSensor_Enhanced.vi"("error in (no error)"=w208, "Feedback Device"=w206, "PhoenixMotorControlDevRef"=w207) -> ("PhoenixMotorControlDevRef"=w186:T9)  [unwired: 7 in, 1 out]
      n84 = call "CTRE_Phoenix_MotorControl_ConfigSelectedFeedbackSensor_Enhanced.vi"("error in (no error)"=w236, "Feedback Device"=w234, "PhoenixMotorControlDevRef"=w235) -> ("PhoenixMotorControlDevRef"=w188:T9)  [unwired: 7 in, 1 out]
      n85 = call "CTRE_Phoenix_MotorControl_Follow.vi"("error in (no error)"=w193, "Master Controller to Follow"=w188, "PhoenixMotorControlDevRef"=w192) -> ()  [unwired: 7 in, 2 out]
      n86 = call "CTRE_Phoenix_MotorControl_ConfigSelectedFeedbackSensor_Enhanced.vi"("error in (no error)"=w222, "Feedback Device"=w220, "PhoenixMotorControlDevRef"=w221) -> ("PhoenixMotorControlDevRef"=w187:T9)  [unwired: 7 in, 1 out]
      n87 = call "CTRE_Phoenix_MotorControl_ConfigSelectedFeedbackSensor_Enhanced.vi"("error in (no error)"=w250, "Feedback Device"=w248, "PhoenixMotorControlDevRef"=w249) -> ("PhoenixMotorControlDevRef"=w189:T9)  [unwired: 7 in, 1 out]
      n88 = call "CTRE_Phoenix_MotorControl_Follow.vi"("error in (no error)"=w200, "Master Controller to Follow"=w189, "PhoenixMotorControlDevRef"=w199) -> ()  [unwired: 7 in, 2 out]
      n89 = call-poly <vilib>:"WPI_RobotDriveOpen4Motor.vi"("Rear Left Motor Dev Ref"=w189, "Rear Right Motor Dev Ref"=w188, "Front Left Motor Dev Ref"=w187, "Front Right Motor Dev Ref"=w186) -> ("RobotDriveDevRef"=w263:T14, "error out"=w262:errorcluster)  [unwired: 10 in]
    }
  }
  n90 = call <vilib>:"WPI_RobotDriveRefNum Registry Set.vi"("error in (no error)"=w8, "refnum name"="Left and Right Motors", "RobotDriveDevRef"=w10) -> ("RobotDriveDevRef"=w7:T14)  [unwired: 1 in, 7 out]
  n91 = call "Drive Controller Initialization.vi"("Subsystem Name"=w11, "Default Command"=w1) -> ("Current Command"=w3:T17)  [unwired: 9 in]
  n92 = call <vilib>:"WPI_RobotDriveSafetyConfig.vi"("mode"=WPI_SafetyOutputConfigMenu."Enable", "RobotDriveDevRef"=w7) -> ("RobotDriveDevRef"=w5:T14)  [unwired: 8 in, 1 out]
  n93 = vi-ref "Reserve Drive.vi"() -> (w2:refnum<vi>)
  n94 = while {
    shift-right: [w271] -> _
    shift-left: w3 -> [w264]
    tunnel: [w283] -> _
    tunnel: w5 -> [w279]
    tunnel: "error in" -> [_]
    tunnel: w2 -> [_]
    i -> [w283]
    stop <- FALSE stop-if-true
    (unwired) "RobotDrive Motors" ("Name")
    # "Step 5: Upate your I/O"
    # "Step 4: Format a string to describe this\ncmd and how the previous cmd finished"
    # "Current Command"
    # "Update motors and update dashboard"
    # "Plot the Setpoints"
    # "Access Cmd setpoints"
    # "Finished? &\nWait Time"
    # "Step 3: For a given operation, read from sensors, perform calculations,\nupdate actuators and status.\nOperations can be merged to a single case."
    n95 = Unbundle(w264) -> ("SubSystem Data"=w278:T1, w265:cluster{"Start Time (ms)":u32, "Iterations":i32})  [unwired: 1 out]
    n96 = Unbundle By Name(w278) -> ("Operation"=w277:T2, "Left Setpoint"=w276:dbl, "Right Setpoint"=w275:dbl, "Duration"=w274:dbl)
    n97 = Tick Count (ms)() -> (millisecond timer value=w273:u32)
    n98 = case shown="\"Immediate\", Default" w277 {
      tunnel: [w302 w303 w318] -> w270
      tunnel: [w295 w310 FALSE ("ignore previous (F)")] -> w269
      tunnel: w265 -> [w294 w312 _]
      tunnel: [w301 w309 w316] -> w281
      tunnel: [w300 w308 w316] -> w280
      tunnel: w276 -> [w301 w309 _]
      tunnel: w275 -> [w300 w308 _]
      tunnel: w274 -> [_ w307 _]
      tunnel: w273 -> [w296 w306 _]
      frame "Immediate", Default {
        w302 = 100.0  # Wait ms
        # "Set motor values for ~50ms. Finish, and reserve, if\nwe exceed that time. This is  to deal with Safety and\njoystick deadband."
        n99 = Unbundle(w294) -> ("Start Time (ms)"=w297:u32)  [unwired: 1 out]
        n100 = Subtract(x=w296, y=w297) -> (x-y=w298:u32)
        n101 = Greater?(x=w298, y=u8 50 ("Left Motor")) -> (0:w295:bool)
      }
      frame "Drive for Time" {
        # "How much longer?\nUpdate motors every 50ms to\nkeep Safety happy"
        n102 = Unbundle(w312) -> ("Start Time (ms)"=w311:u32)  [unwired: 1 out]
        n103 = Subtract(x=w306, y=w311) -> (x-y=w315:u32)
        n104 = Multiply(x=w307, y=1000.0) -> (x*y=w314:dbl)
        n105 = Subtract(x=w314, y=w315) -> (x-y=w305:dbl)
        n106 = Less Or Equal To 0?(x=w305) -> (x <= 0?=w310:bool)
        n107 = Max & Min(x=w305, y=50.0) -> (min(x,y)=w303:dbl)  [unwired: 1 out]
      }
      frame "Reserve" {
        w316 = 0.0  # Don't move motors while reserved
        w318 = -1.0  # Infinite
        # "If loop needs to poll sensors or other\nvalues, use a timeout value. -1 waits for\nnext command to be sent."
      }
    }
    n108 = call "Drive Check for New Command.vi"("input cluster"=w264, "Wait time (ms)"=w270, "Finished?"=w269) -> ("Completion"=w272:T3, "Subsystem Name"=w266:string, "Current Command"=w267:T1, "Initial Trace String"=w268:string, "Next Command"=w271:T18)  [unwired: 4 in]
    n109 = Bundle("Don't move motors while reserved"=w281, "Don't move motors while reserved"=w280) -> (→"Setpoints":T19)  [unwired: 1 in]
    n110 = call <vilib>:"WPI_RobotDriveMotors.vi"("RightSpeed"=w280, "LeftSpeed"=w281, "RobotDriveDevRef"=w279) -> ()  [unwired: 1 in, 8 out]
    n111 = case shown="\"Successful\", \"Aborted\"" w272 {
      selector: w272 -> [_ w293]
      tunnel: w268 -> [_ w288]
      tunnel: w267 -> [_ w289]
      tunnel: w266 -> [_ w285]
      frame "Incomplete", Default {
        # "Continuing current command"
      }
      frame "Successful", "Aborted" {
        # "Report and setup for next command"
        n112 = Unbundle By Name(w289) -> ("Left Setpoint"=w291:dbl, "Right Setpoint"=w292:dbl, "Duration"=w286:dbl)
        n113 = Format Into String(format string="L %.1f, R %.1f, D %f", initial string=w288, w291, w292, w286) -> (resulting string=w287:string)  [unwired: 1 in, 1 out]
        "Current\nCmd" <- w287
        n114 = call <vilib>:"Trace Results.vi"("Status of previous command"=w293, "Description"=w287, "Subsystem"=w285) -> ()  [unwired: 9 in]
      }
    }
  }
  n115 = while {
    tunnel: w1 -> [w320]
    stop <- FALSE stop-if-true
    n116 = call "Drive Controller Interactive Check.vi"("Interactive Command In"="Interactive Values", "Default Command"=w320, "Buttons"="Buttons") -> ("Interactive Command Out"=w322:T1, "Trace String"=w323:string, "Schedule"=w324:bool)  [unwired: 6 in]
    n117 = case shown="True" w324 {
      tunnel: [w333 w341] -> w325
      tunnel: [w332 w337] -> w326
      tunnel: w323 -> [_ w339]
      tunnel: w322 -> [_ w338]
      frame False {
        n118 = Tick Count (ms)() -> (millisecond timer value=w336:u32)
        n119 = call "Read Drive Operation.vi"() -> ("Command Info"=w330:T15, "SubSystem Data"=w329:T1)  [unwired: 9 in, 1 out]
        n120 = Unbundle(w329) -> ("Operation"=w334:T2, "Left Setpoint"=w331:dbl)  [unwired: 2 out]
        n121 = Unbundle(w330) -> ("Status"=w333:T3)  [unwired: 2 out]
        n122 = Subtract(x=w336, y=w334) -> (x-y=w335:u32)
        n123 = Bundle(w335, "Left Setpoint"=w331) -> (w332:cluster{u32, "Left Setpoint":dbl})  [unwired: 1 in]
      }
      frame True {
        n124 = call "Drive Command Helper.vi"("Description"=w339, "SubSystem Data"=w338) -> ("Command Info Out"=w340:T15, "Command Timing"=w337:cluster{"Start Time (ms)":u32, "Iterations":i32})  [unwired: 7 in, 1 out]
        n125 = Unbundle(w340) -> ("Status"=w341:T3)  [unwired: 2 out]
      }
    }
    "Status" <- w325
    "Command Timing" <- w326
    n126 = Wait (ms)(milliseconds to wait=u32 20) -> ()  [unwired: 1 out]
  }
